vi "Get Template Size.vi"(8 "error in (no error)":errorcluster, 11 "Control in":refnum<class "Control.lvclass">) -> (0 "error out":errorcluster, 2 "Button Size":cluster{"Width":i32, "Height":i32} caption="Size", 3 "Control out":refnum<class "Control.lvclass">)   [LabVIEW 2013, in "uitools_Control.lvlib" / "Control.lvclass"]
uses:
  Control.lvclass
  <userlib>/BitMan/BitMap class/BitMap.lvclass
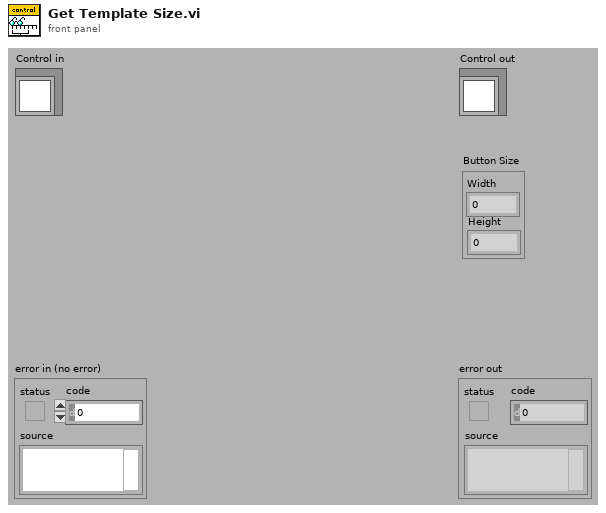
[diagram p1: front panel]
types:
  T1 = typedef "imagedata.ctl" = cluster{"image type":i32, "image depth":i32, "image":u8[], "mask":u8[], "colors":u32[], "Rectangle":cluster{"left":i16, "top":i16, "right":i16, "bottom":i16}}
  T2 = typedef "BitMan Lib.lvlib/Size type.ctl" = cluster{"Width":i32, "Height":i32}
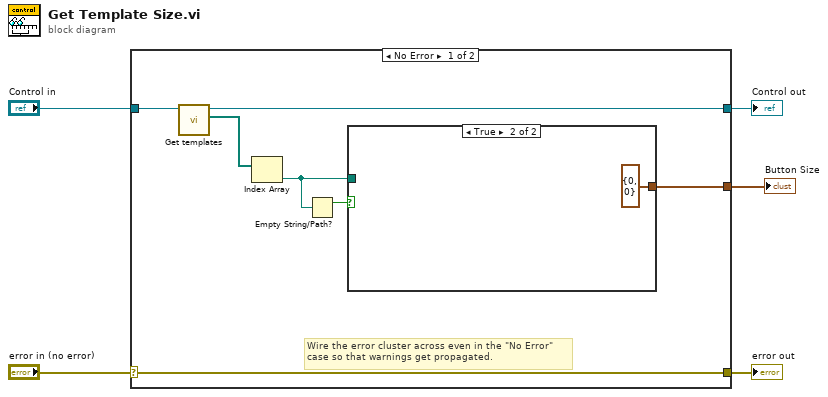
[diagram p0: block diagram]
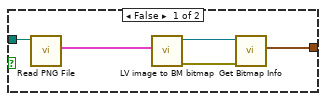
[diagram p2: hidden frame]
diagram:
  n1 = case shown="No Error" "error in (no error)" {
    selector: "error in (no error)" -> [w12 w20]
    tunnel: [w12 w20] -> w4
    tunnel: [w9 w19] -> w2
    tunnel: "Control in" -> [w10 w19]
    tunnel: [w11 _] -> w1
    frame No Error {
      # "Wire the error cluster across even in the \"No Error\"\ncase so that warnings get propagated."
      n2 = call-dynamic "Get templates.vi"("Control in"=w10) -> ("PNG templates"=w8:path[], "Control out"=w9:refnum<class "Control.lvclass">)  [unwired: 1 in, 8 out]
      n3 = Index Array(array=w8) -> (element=w7:path)  [unwired: 1 in]
      n4 = Empty String/Path?(string/path=w7) -> (empty?=w6:bool)
      n5 = case shown="True" w6 {
        tunnel: [w17 cluster{"Width":i32, "Height":i32} {"Width"=0, "Height"=0} ("Size")] -> w11
        tunnel: w7 -> [w14 _]
        frame False {
          n6 = call <vilib>:"Read PNG File.vi"("path to PNG file"=w14) -> ("image data"=w15:T1)  [unwired: 1 in, 9 out]
          n7 = call <userlib>:"LV image to BM bitmap.vi"("LV image data"=w15) -> ("error out"=w13:errorcluster, "BitMap out"=w16:refnum<class "BitMap.lvclass">)  [unwired: 3 in, 6 out]
          n8 = call <userlib>:"Get Bitmap Info.vi"("error in (no error)"=w13, "BitMap in"=w16) -> ("Size"=w17:T2)  [unwired: 9 out]
        }
        frame True {
        }
      }
    }
    frame Error {
    }
  }
  "error out" <- w4
  "Control out" <- w2
  "Button Size" <- w1
